vi "test get from map as type.vi"() -> (1 "pass?":bool)   [LabVIEW 2019, in "LVCOOOP Tests.lvlib"]
uses:
  LVCOOOP Tests.lvlib
  b7fdc737-810d-476c-803f-87d92304fadd.vi
  7fb67aad-f021-4248-8772-102f8fa4be12.vi
  03525885-fed1-44f0-abe8-b2b06852e5b1.vi
  eb1a332b-77f4-454b-9d65-ac763f45a6a6.vi
  6fdd71bf-bd25-4e1a-bc78-942183a96767.vi
  209f202e-6f5e-4ae7-91fa-58a3fdf974fc.vi
  15cceecd-e535-48b2-a859-5fa44f02509e.vi
  98d83769-089f-491f-aeb6-b46676a4fedc.vi
  b7fdc737-810d-476c-803f-87d92304fadd.vi/aefe0d59-7504-4126-851e-01b31108fa54.vi
  7fb67aad-f021-4248-8772-102f8fa4be12.vi/e3f2c800-51ad-42b8-aec2-43565a1109b2.vi
  7fb67aad-f021-4248-8772-102f8fa4be12.vi/316e8c77-036e-4d79-b6d4-aae30502cda3.vi
  03525885-fed1-44f0-abe8-b2b06852e5b1.vi/d39bf774-7627-41f1-aaab-c2a36143d0c8.vi
  03525885-fed1-44f0-abe8-b2b06852e5b1.vi/6db067e0-832c-4795-8ece-8102970040d3.vi
  eb1a332b-77f4-454b-9d65-ac763f45a6a6.vi/430bb046-5b81-413a-9df3-69019fa30a5d.vi
  eb1a332b-77f4-454b-9d65-ac763f45a6a6.vi/91dc9289-ab46-4558-b6da-fda84c024f8f.vi
  6fdd71bf-bd25-4e1a-bc78-942183a96767.vi/6e523f6e-8c07-4574-88fa-9a46ce79b174.vi
  6fdd71bf-bd25-4e1a-bc78-942183a96767.vi/872a4fc2-fcd1-4935-a799-567209630bc0.vi
  209f202e-6f5e-4ae7-91fa-58a3fdf974fc.vi/df1c9b35-4c63-4de3-96a4-fc5ec339da08.vi
  15cceecd-e535-48b2-a859-5fa44f02509e.vi/43c71af7-87af-4bf9-964d-8e9921bd185c.vi
  15cceecd-e535-48b2-a859-5fa44f02509e.vi/1af4038f-45b9-4805-99bf-4316df907d14.vi
  98d83769-089f-491f-aeb6-b46676a4fedc.vi/b919ee37-8e9f-42a1-afca-5b3730f5890a.vi
  98d83769-089f-491f-aeb6-b46676a4fedc.vi/bbf8bb24-86b2-4b03-94f3-ba8412c5f0cd.vi
panel:
  out "int arry pass?":bool
  out "sgl arry pass?":bool
  out "path pass?":bool
  out "U64 pass?":bool
  out "I32 pass?":bool
  out "U32 pass?":bool
  out "double pass?":bool
  out "string pass?":bool
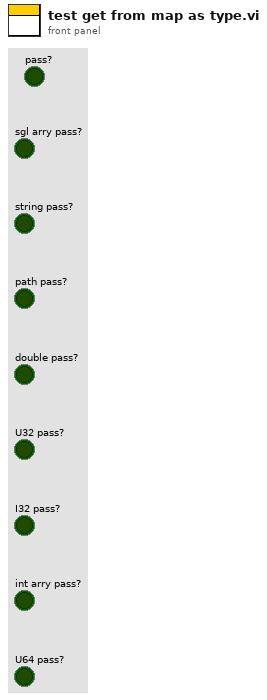
[diagram p1: front panel]
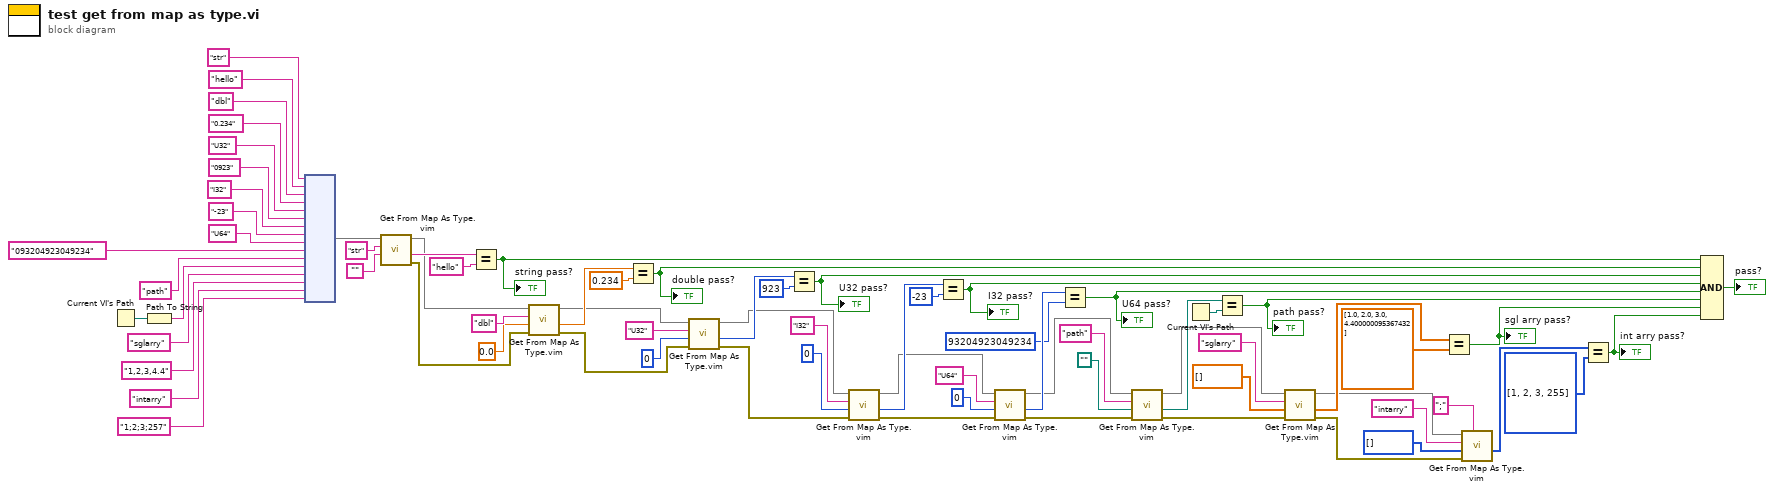
[diagram p0: block diagram]
diagram:
  n1 = Current VI's Path() -> (path=w63:path)
  n2 = Path To String(path=w63) -> (string=w62:string)
  n3 = node("str", "hello", "dbl", "0.234", "U32", "0923", "I32", "-23", "U64", "093204923049234", "path", w62, "sglarry", "1,2,3,4.4", "intarry", "1;2;3;257") -> (w57:map{string, string})
  n4 = call "Get From Map As Type.vim"("default"="", "key"="str", "map in"=w57) -> ("error out"=w22:errorcluster, "value"=w54:string, "map out (unchanged)"=w52:map{string, string})  [unwired: 5 in, 1 out]
  n5 = Equal?(x=w54, y="hello") -> (x = y?=w9:bool)
  "string pass?" <- w9
  n6 = call "Get From Map As Type.vim"("error in (no error)"=w22, "default"=0.0, "key"="dbl", "map in"=w52) -> ("error out"=w21:errorcluster, "value"=w49:dbl, "map out (unchanged)"=w44:map{string, string})  [unwired: 4 in, 1 out]
  n7 = Equal?(x=w49, y=0.234) -> (x = y?=w8:bool)
  "double pass?" <- w8
  n8 = call "Get From Map As Type.vim"("error in (no error)"=w21, "default"=u32 0 ("y"), "key"="U32", "map in"=w44) -> ("error out"=w20:errorcluster, "value"=w46:u32, "map out (unchanged)"=w38:map{string, string})  [unwired: 4 in, 1 out]
  n9 = Equal?(x=w46, y=u32 923) -> (x = y?=w7:bool)
  "U32 pass?" <- w7
  n10 = call "Get From Map As Type.vim"("error in (no error)"=w20, "default"=0 ("y"), "key"="I32", "map in"=w38) -> ("error out"=w19:errorcluster, "value"=w41:i32, "map out (unchanged)"=w33:map{string, string})  [unwired: 4 in, 1 out]
  n11 = Equal?(x=w41, y=-23) -> (x = y?=w6:bool)
  "I32 pass?" <- w6
  n12 = call "Get From Map As Type.vim"("error in (no error)"=w19, "default"=u64 0 ("y"), "key"="U64", "map in"=w33) -> ("error out"=w18:errorcluster, "value"=w35:u64, "map out (unchanged)"=w32:map{string, string})  [unwired: 4 in, 1 out]
  n13 = Equal?(x=w35, y=u64 93204923049234) -> (x = y?=w5:bool)
  "U64 pass?" <- w5
  n14 = call "Get From Map As Type.vim"("error in (no error)"=w18, "default"=path "", "key"="path", "map in"=w32) -> ("error out"=w17:errorcluster, "value"=w29:path, "map out (unchanged)"=w27:map{string, string})  [unwired: 4 in, 1 out]
  n15 = Current VI's Path() -> (path=w28:path)
  n16 = Equal?(x=w29, y=w28) -> (x = y?=w4:bool)
  "path pass?" <- w4
  n17 = call "Get From Map As Type.vim"("error in (no error)"=w17, "default"=sgl[] [], "key"="sglarry", "map in"=w27) -> ("error out"=w16:errorcluster, "value"=w24:sgl[], "map out (unchanged)"=w15:map{string, string})  [unwired: 4 in, 1 out]
  n18 = Equal?(x=w24, y=sgl[] [1.0, 2.0, 3.0, 4.4]) -> (x = y?=w3:bool)
  "sgl arry pass?" <- w3
  n19 = call "Get From Map As Type.vim"("array delimeter (,)"=";", "error in (no error)"=w16, "default"=u8[] [], "key"="intarry", "map in"=w15) -> ("value"=w11:u8[])  [unwired: 3 in, 3 out]
  n20 = Equal?(x=w11, y=u8[] [1, 2, 3, 255]) -> (x = y?=w2:bool)
  "int arry pass?" <- w2
  n21 = Compound Arithmetic op=AND(w9, w8, w7, w6, w5, w4, w3, w2) -> (→"pass?":bool)
